vi "Create Receive Thread.vi"(11 "OpenStatus":bool) -> ()   [LabVIEW 2011, in "CAN FD.lvlib"]
uses:
  CAN FD.lvlib
  Receive Thread.vi
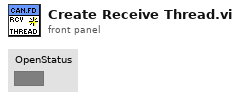
[diagram p1: front panel]
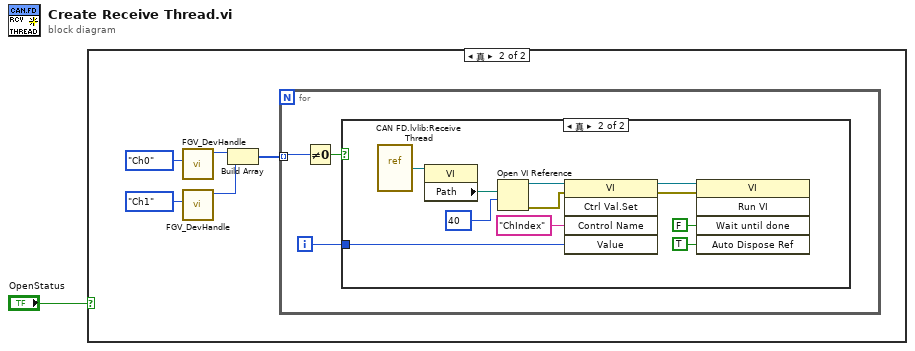
[diagram p0: block diagram]
diagram:
  n1 = case shown="真" "OpenStatus" {
    frame False {
    }
    frame True {
      n2 = call "FGV_DevHandle.vi"("Type"=enum16{"Device", "Ch0", "Ch1"}."Ch0") -> ("handle out"=w4:u32)  [unwired: 8 in, 2 out]
      n3 = call "FGV_DevHandle.vi"("Type"=enum16{"Device", "Ch0", "Ch1"}."Ch1") -> ("handle out"=w3:u32)  [unwired: 8 in, 2 out]
      n4 = Build Array(w4, w3) -> (w2:u32[])
      n5 = for {
        tunnel: w2 -> [w9] mode=indexing
        i -> [w7]
        n6 = Not Equal To 0?(x=w9) -> (x != 0?=w8:bool)
        n7 = case shown="真" w8 {
          tunnel: w7 -> [_ w15]
          frame False {
          }
          frame True {
            n8 = vi-ref "CAN FD.lvlib:Receive Thread.vi"() -> (w20:refnum<vi>)
            n9 = property class="VI"(reference=w20) -> ("Path"=w19:path)  [unwired: 1 in, 2 out]
            n10 = Open VI Reference(vi path=w19, options=40 ("选项")) -> (vi reference=w17:refnum<vi>, error out=w14:errorcluster)  [unwired: 4 in]
            n11 = invoke class="VI" method="Ctrl Val.Set"(reference=w17, error in=w14, "Control Name"="ChIndex" ("控件名"), "Value"=w15) -> (reference out=w13:refnum<vi>, error out=w12:errorcluster)  [unwired: 1 in, 3 out]
            n12 = invoke class="VI" method="Run VI"(reference=w13, error in=w12, "Wait until done"=FALSE ("结束前等待"), "Auto Dispose Ref"=TRUE ("自动销毁引用")) -> ()  [unwired: 1 in, 5 out]
          }
        }
      }
    }
  }
